vi "FGV_Initialization.vi"(8 "error in (no error)":errorcluster) -> (0 "error out":errorcluster)   [LabVIEW 2025]
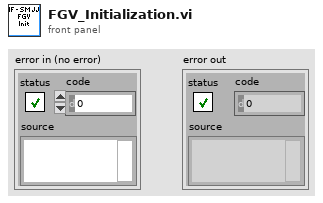
[diagram p1: front panel]
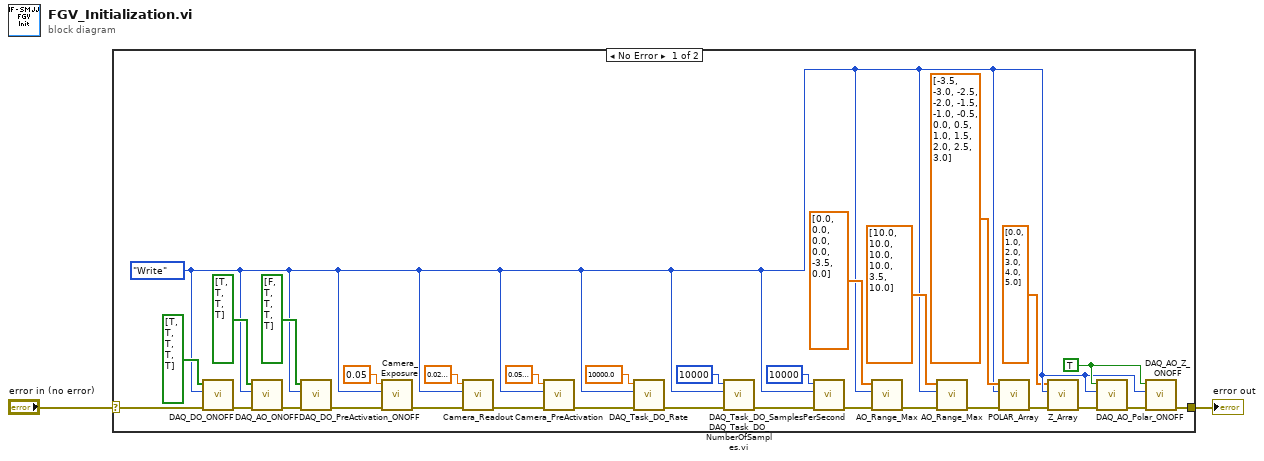
[diagram p0: block diagram]
diagram:
  n1 = case shown="No Error" "error in (no error)" {
    selector: "error in (no error)" -> [w25 w34]
    tunnel: [w7 w34] -> w2
    frame No Error {
      w9 = TRUE ("ON / OFF")
      w4 = enum16{"Write", "Read"}."Write" ("Action")
      n2 = call "DAQ_DO_ONOFF.vi"("error in"=w25, "Action"=w4, "DO | ON/OFF"=bool[] [TRUE, TRUE, TRUE, TRUE, TRUE]) -> ("error out"=w17:errorcluster)  [unwired: 7 in, 1 out]
      n3 = call "DAQ_AO_ONOFF.vi"("error in"=w17, "Action"=w4, "AO | ON/OFF"=bool[] [TRUE, TRUE, TRUE, TRUE]) -> ("error out"=w16:errorcluster)  [unwired: 7 in, 1 out]
      n4 = call "DAQ_DO_PreActivation_ONOFF.vi"("error in"=w16, "Action"=w4, "DO | PreActivation ON/OFF"=bool[] [FALSE, TRUE, TRUE, TRUE, TRUE] ("DO | PreActivation")) -> ("error out"=w33:errorcluster)  [unwired: 7 in, 1 out]
      n5 = call "Camera_Exposure.vi"("error in"=w33, "Action"=w4, "Exposure (s)"=0.05 ("Exposure time (s)")) -> ("error out"=w29:errorcluster)  [unwired: 7 in, 1 out]
      n6 = call "Camera_Readout.vi"("error in"=w29, "Action"=w4, "Camera_Readout"=0.020000000000000018 ("Readout time (s)")) -> ("error out"=w31:errorcluster)  [unwired: 7 in, 1 out]
      n7 = call "Camera_PreActivation.vi"("error in"=w31, "Action"=w4, "Camera_PreActivation"=0.050000000000000044 ("Pre-activation time (s)")) -> ("error out"=w23:errorcluster)  [unwired: 7 in, 1 out]
      n8 = call "DAQ_Task_DO_Rate.vi"("error in"=w23, "Action"=w4, "DO_Rate"=10000.0) -> ("error out"=w24:errorcluster)  [unwired: 7 in, 1 out]
      n9 = call "DAQ_Task_DO_NumberOfSamples.vi.vi"("error in"=w24, "Action"=w4, "Samples"=10000) -> ("error out"=w20:errorcluster)  [unwired: 7 in, 1 out]
      n10 = call "DAQ_Task_DO_SamplesPerSecond.vi"("error in"=w20, "Action"=w4, "DO_Task_SamplesPerSec"=u32 10000) -> ("error out"=w12:errorcluster)  [unwired: 7 in, 1 out]
      n11 = call "AO_Range_Max.vi"("error in"=w12, "Action"=w4, "AO | Max"=dbl[] [0.0, 0.0, 0.0, 0.0, -3.5, 0.0]) -> ("error out"=w11:errorcluster)  [unwired: 7 in, 1 out]
      n12 = call "AO_Range_Max.vi"("error in"=w11, "Action"=w4, "AO | Max"=dbl[] [10.0, 10.0, 10.0, 10.0, 3.5, 10.0]) -> ("error out"=w14:errorcluster)  [unwired: 7 in, 1 out]
      n13 = call "POLAR_Array.vi"("error in"=w14, "Action"=w4, "Pockels_Array"=dbl[] [-3.5, -3.0, -2.5, -2.0, -1.5, -1.0, -0.5, 0.0, 0.5, 1.0, 1.5, 2.0, 2.5, 3.0]) -> ("error out"=w6:errorcluster)  [unwired: 7 in, 1 out]
      n14 = call "Z_Array.vi"("error in"=w6, "Action"=w4, "Z Array"=dbl[] [0.0, 1.0, 2.0, 3.0, 4.0, 5.0]) -> ("error out"=w5:errorcluster)  [unwired: 7 in, 1 out]
      n15 = call "DAQ_AO_Polar_ONOFF.vi"("error in"=w5, "Action"=w4, "ON / OFF"=w9) -> ("error out"=w8:errorcluster)  [unwired: 7 in, 1 out]
      n16 = call "DAQ_AO_Z_ONOFF.vi"("error in"=w8, "Action"=w4, "ON / OFF"=w9) -> ("error out"=w7:errorcluster)  [unwired: 7 in, 1 out]
    }
    frame Error {
    }
  }
  "error out" <- w2
